vi "producer-consumer.vi"() -> ()   [LabVIEW 2023]
uses:
  Control Timer.ctl
panel:
  out "State":string
  out "error out":errorcluster
  out "Diode":bool
  in  "stop":bool
  in  "Test 2":bool
  in  "Test 1":bool
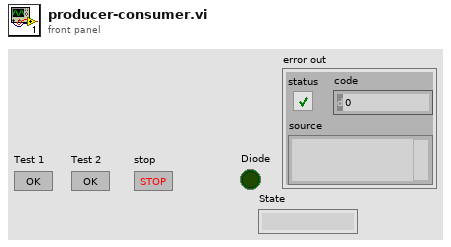
[diagram p1: front panel]
types:
  T1 = typedef "Control Timer.ctl" = enum16{"Timecheck", "Reset"}
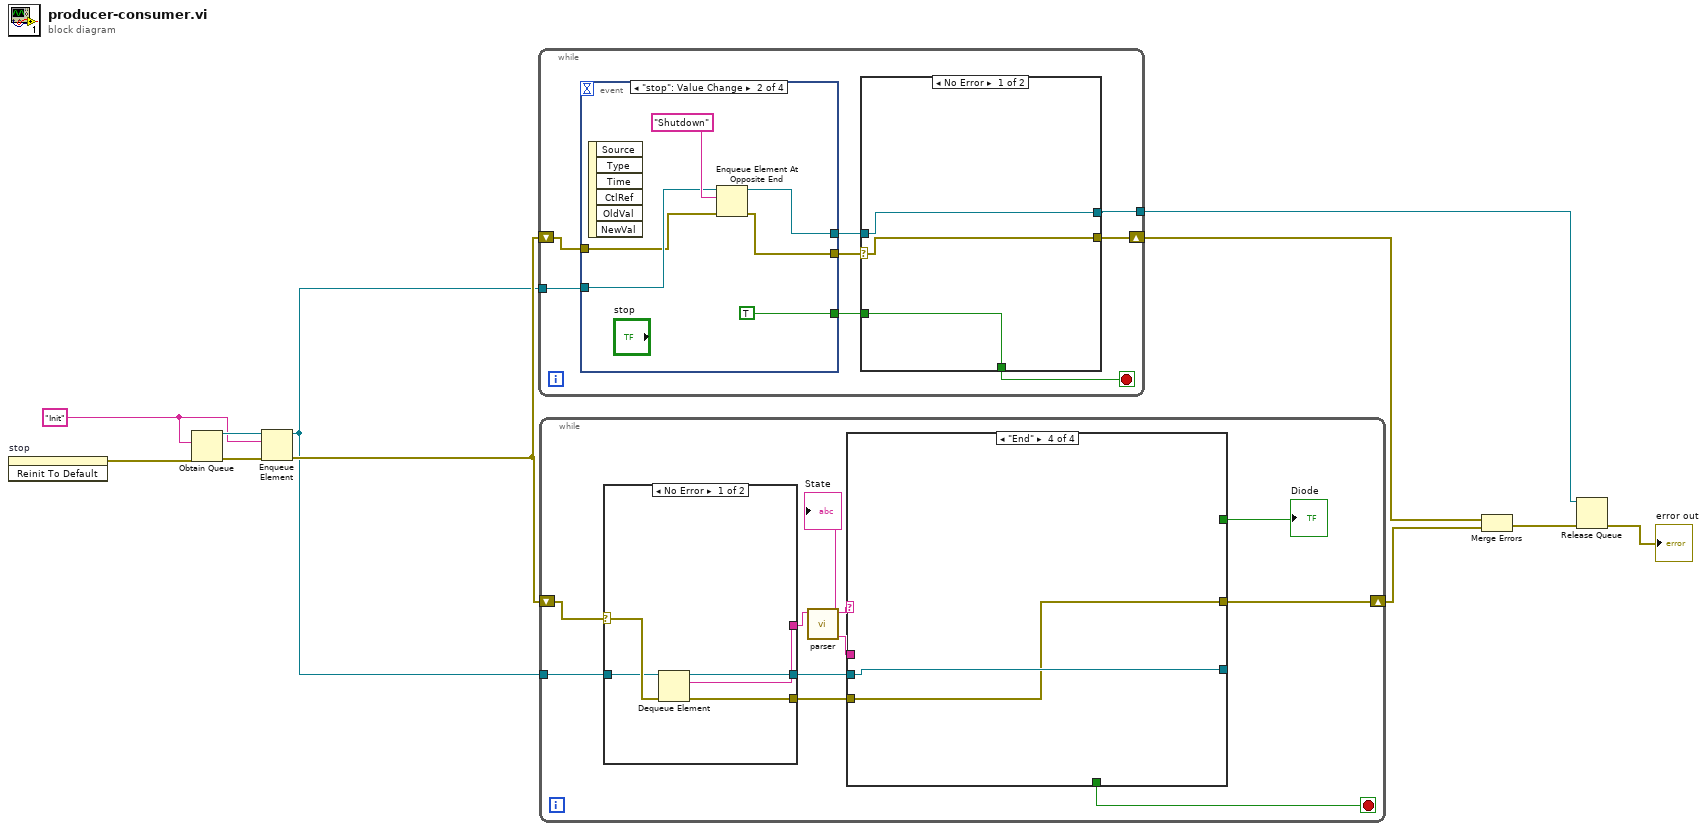
[diagram p0: block diagram]
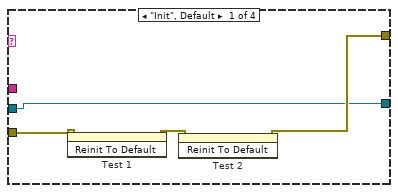
[diagram p2: hidden frame]
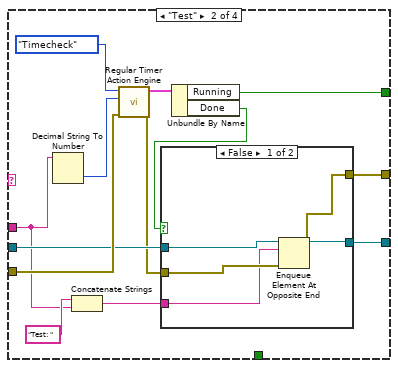
[diagram p3: hidden frame]
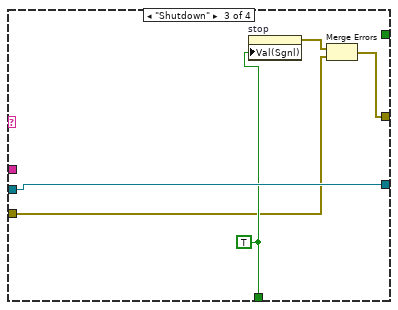
[diagram p5: hidden frame]
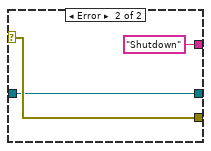
[diagram p6: hidden frame]
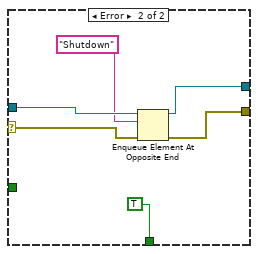
[diagram p7: hidden frame]
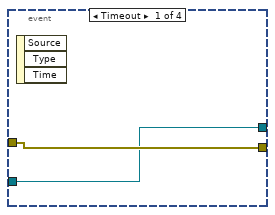
[diagram p8: hidden frame]
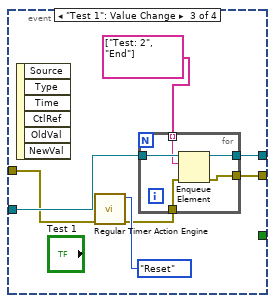
[diagram p9: hidden frame]
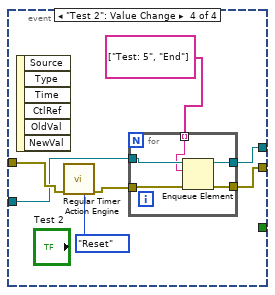
[diagram p10: hidden frame]
diagram:
  w9 = "Init"
  n1 = invoke on="stop" class="Bool (strict)" method="Reinit To Default"() -> (error out=w11:errorcluster)  [unwired: 3 in, 2 out]
  n2 = Obtain Queue(element data type=w9, error in (no error)=w11) -> (queue out=w10:refnum<queue>, error out=w8:errorcluster)  [unwired: 3 in, 1 out]
  n3 = Enqueue Element(queue=w10, element=w9, error in (no error)=w8) -> (queue out=w6:refnum<queue>, error out=w7:errorcluster)  [unwired: 1 in, 1 out]
  n4 = while {
    tunnel: w6 -> [w19]
    shift-right: [w15] -> w4
    shift-left: w7 -> [w17]
    tunnel: [w14] -> w2
    stop <- w13 stop-if-true
    n5 = event shown="[1] \"stop\": Value Change" {
      selector: _ -> [_ _ _ _]
      dyn-events: _ -> [_ _ _ _]
      timeout: _ -> [_ _ _ _]
      tunnel: w19 -> [w29 w35 w43 w51]
      tunnel: [w30 w34 w37 w50] -> w18
      tunnel: w17 -> [w30 w33 w40 w55]
      tunnel: [w29 w32 w41 w49] -> w16
      tunnel: [_ TRUE _ _] -> w12
      event Timeout {
        n6 = event-data() -> ()  [unwired: 1 in, 3 out]
      }
      event "stop": Value Change {
        n7 = event-data() -> ()  [unwired: 1 in, 6 out]
        n8 = Enqueue Element At Opposite End(queue=w35, element="Shutdown", error in (no error)=w33) -> (queue out=w32:refnum<queue>, error out=w34:errorcluster)  [unwired: 1 in, 1 out]
      }
      event "Test 1": Value Change {
        n9 = event-data() -> ()  [unwired: 1 in, 6 out]
        n10 = call "Regular Timer Action Engine.vi"("Enum"=Control_Timer."Reset", "error in"=w40) -> ("error out"=w38:errorcluster)  [unwired: 7 in, 1 out]
        n11 = for {
          tunnel: w43 -> [w48]
          tunnel: string[] ["Test: 2", "End"] -> [w47] mode=indexing
          tunnel: [w46] -> w41
          tunnel: w38 -> [w45]
          tunnel: [w44] -> w37
          n12 = Enqueue Element(queue=w48, element=w47, error in (no error)=w45) -> (queue out=w46:refnum<queue>, error out=w44:errorcluster)  [unwired: 1 in, 1 out]
        }
      }
      event "Test 2": Value Change {
        n13 = event-data() -> ()  [unwired: 1 in, 6 out]
        n14 = call "Regular Timer Action Engine.vi"("Enum"=Control_Timer."Reset", "error in"=w55) -> ("error out"=w53:errorcluster)  [unwired: 7 in, 1 out]
        n15 = for {
          tunnel: w53 -> [w58]
          tunnel: string[] ["Test: 5", "End"] -> [w59] mode=indexing
          tunnel: w51 -> [w60]
          tunnel: [w57] -> w50
          tunnel: [w56] -> w49
          n16 = Enqueue Element(queue=w60, element=w59, error in (no error)=w58) -> (queue out=w56:refnum<queue>, error out=w57:errorcluster)  [unwired: 1 in, 1 out]
        }
      }
    }
    n17 = case shown="No Error" w18 {
      selector: w18 -> [w22 w28]
      tunnel: w16 -> [w21 w26]
      tunnel: [w22 w27] -> w15
      tunnel: [w21 w25] -> w14
      tunnel: [w20 TRUE] -> w13
      tunnel: w12 -> [w20 _]
      frame No Error {
      }
      frame Error {
        n18 = Enqueue Element At Opposite End(queue=w26, element="Shutdown", error in (no error)=w28) -> (queue out=w25:refnum<queue>, error out=w27:errorcluster)  [unwired: 1 in, 1 out]
      }
    }
  }
  n19 = while {
    shift-right: [w64] -> w5
    shift-left: w7 -> [w70]
    tunnel: w6 -> [w69]
    stop <- w61 stop-if-true
    n20 = case shown="No Error" w70 {
      selector: w70 -> [w106 w108]
      tunnel: [w105 "Shutdown"] -> w68
      tunnel: w69 -> [w104 w107]
      tunnel: [w103 w108] -> w65
      tunnel: [w102 w107] -> w62
      frame No Error {
        n21 = Dequeue Element(queue=w104, error in (no error)=w106) -> (queue out=w102:refnum<queue>, element=w105:string, error out=w103:errorcluster)  [unwired: 1 in, 1 out]
      }
      frame Error {
      }
    }
    n22 = call "parser.vi"("Input"=w68) -> ("Argument"=w66:string, "State"=w67:string)  [unwired: 9 in]
    "State" <- w67
    n23 = case shown="\"End\"" w67 {
      tunnel: w66 -> [_ w79 _ _]
      tunnel: w65 -> [w74 w82 w97 w100]
      tunnel: [w72 w76 w95 w100] -> w64
      tunnel: [_ w84 _ _] -> w63
      tunnel: w62 -> [w71 w81 w99 w101]
      tunnel: [w71 w75 w99 w101] -> _
      tunnel: [_ _ w98 _] -> w61
      frame "Init", Default {
        n24 = invoke on="Test 1" class="Bool" method="Reinit To Default"(error in=w74) -> (error out=w73:errorcluster)  [unwired: 2 in, 2 out]
        n25 = invoke on="Test 2" class="Bool" method="Reinit To Default"(error in=w73) -> (error out=w72:errorcluster)  [unwired: 2 in, 2 out]
      }
      frame "Test" {
        n26 = Decimal String To Number(string=w79) -> (number=w86:i32)  [unwired: 2 in, 1 out]
        n27 = Concatenate Strings("Test: " ("string"), w79) -> (w78:string)
        n28 = call "Regular Timer Action Engine.vi"("Enum"=Control_Timer."Timecheck", "Time Target"=w86, "error in"=w82) -> ("Status"=w85:cluster{"Running":bool, "Done":bool}, "error out"=w77:errorcluster)  [unwired: 6 in]
        n29 = Unbundle By Name(w85) -> ("Running"=w84:bool, "Done"=w83:bool)
        n30 = case shown="False" w83 {
          tunnel: w81 -> [w91 w93]
          tunnel: w78 -> [w90 _]
          tunnel: w77 -> [w92 w94]
          tunnel: [w89 w94] -> w76
          tunnel: [w88 w93] -> w75
          frame False {
            n31 = Enqueue Element At Opposite End(queue=w91, element=w90, error in (no error)=w92) -> (queue out=w88:refnum<queue>, error out=w89:errorcluster)  [unwired: 1 in, 1 out]
          }
          frame True {
          }
        }
      }
      frame "Shutdown" {
        w98 = TRUE
        n32 = property on="stop" class="Bool (strict)"("Val(Sgnl)"=w98) -> (error out=w96:errorcluster)  [unwired: 2 in, 1 out]
        n33 = Merge Errors(w96, w97) -> (w95:errorcluster)
      }
      frame "End" {
      }
    }
    "Diode" <- w63
  }
  n34 = Merge Errors(w4, w5) -> (w3:errorcluster)
  n35 = Release Queue(queue=w2, error in (no error)=w3) -> (error out=→"error out":errorcluster)  [unwired: 1 in, 2 out]
